vi "Re-init.vi"(6 "instVIref":T1, 8 "tsRef":refnum<vi>, 11 "target in":refnum<class "RTTarget.lvclass">) -> (0 "tsRef out":refnum<vi>, 3 "target out":refnum<class "Base Target.lvclass">)   [LabVIEW 2020, in "NI_TargetHelper.lvlib" / "RTTarget.lvclass"]
uses:
  <vilib>/TargetSupport/NI_TargetHelper/RTTarget/RTTarget.lvclass
  e:/builds/penguin/labview/branches/2020/dev/dist/vi.lib/TargetSupport/NI_TargetHelper/Base Target/Base Target.lvclass
  <vilib>/TargetSupport/NI_TargetHelper/Base Target/Base Target.lvclass
  <vilib>/TargetSupport/NI_TargetHelper/Instance VIref.ctl
  <vilib>/TargetSupport/NI_TargetHelper/NI_TargetHelper.lvlib
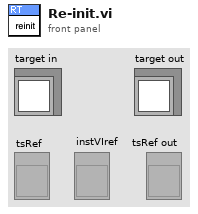
[diagram p1: front panel]
types:
  T1 = typedef "NI_TargetHelper.lvlib/Instance VIref.ctl" = refnum<vi>
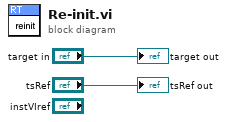
[diagram p0: block diagram]
diagram:
  "target out" <- "target in"
  "tsRef out" <- "tsRef"
